vi "Test_API_InitInvalidInputArraySinks_NoLogger.vi"(8 "error in (no error)":errorcluster, 11 "TestCase in":refnum<class "TestLocalLogInstance.lvclass">) -> (0 "error out":errorcluster, 3 "TestCase out":refnum<class "TestLocalLogInstance.lvclass">)   [LabVIEW 2017, in "TestLocalLogInstance.lvclass"]
uses:
  TestLocalLogInstance.lvclass
  Source/Composed Log/Log Sink/Log Sink.lvclass
  Source/Composed Log/LoggerReference/LoggerReference.lvclass/LoggerReference.ctl
  9a0b009a-159a-478b-8bd0-efcaa49947a6.vi
  Source/Composed Log/LoggerReference/Return Aggregate Queues.vi
  Source/Composed Log/LoggerReference/Add Aggregate Log.vi
  9a0b009a-159a-478b-8bd0-efcaa49947a6.vi/8a2c22db-00e5-40c9-a6c7-b08857810732.vi
  Source/Composed Log/LoggerReference/Log.vi
  Source/Composed Log/LoggerReference/Send Add Sink.vi
  Source/Composed Log/LoggerReference/Remove Stale Logs.vi
  Source/Composed Log/Application Logger/Launch Worker Loop.vi
  Source/Composed Log/LoggerReference/Initialize Logger Instance.vi
  Source/Composed Log/LoggerReference/LoggerReference.lvclass
  Source/Composed Log/IErrorFormat/IErrorFormat.lvclass
  <vilib>/addons/_JKI Toolkits/VI Tester/TestCase.llb/TestCase.lvclass
  C:/Program Files (x86)/National Instruments/LabVIEW 2017/vi.lib/addons/_JKI Toolkits/VI Tester/TestCase.llb/TestCase.lvclass
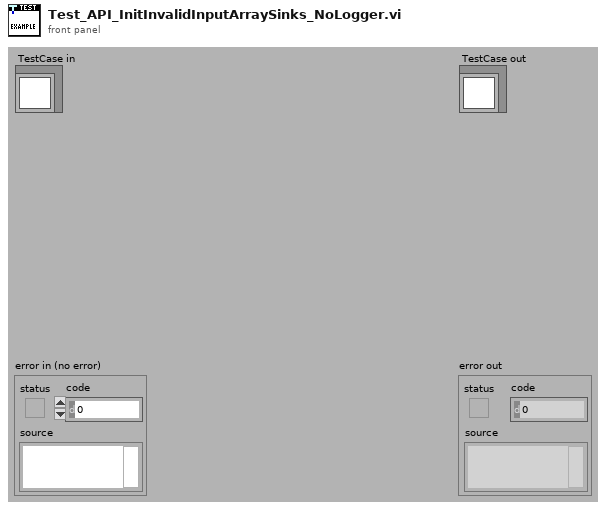
[diagram p1: front panel]
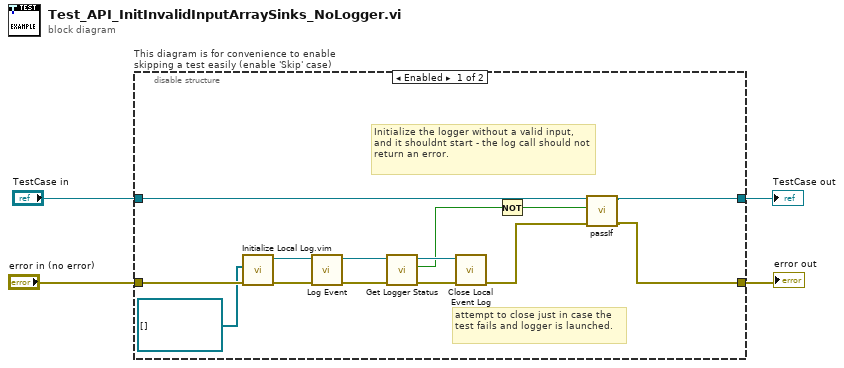
[diagram p0: block diagram]
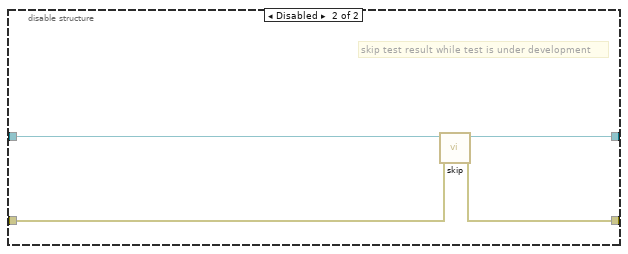
[diagram p2: hidden frame]
diagram:
  n1 = disable-structure "This diagram is for convenience to enable skipping a test easily (enable 'Skip' case)" shown="Enabled" {
    disable-tunnel: "TestCase in" -> [w12 w22]
    disable-tunnel: [w11 w20] -> w1
    disable-tunnel: [w14 w21] -> w3
    disable-tunnel: "error in (no error)" -> [w18 w19]
    frame Enabled {
      # "attempt to close just in case the test fails and logger is launched."
      # "Initialize the logger without a valid input, and it shouldnt start - the log call should not return an error."
      n2 = call "Initialize Local Log.vim"("error in (no error)"=w18, "Startup Sink(s)"=refnum<class "Log Sink.lvclass">[] [] ("Log Sink")) -> ("error out"=w17:errorcluster, "Log Instance Reference"=w16:refnum<class "LoggerReference.lvclass">)  [unwired: 7 in, 1 out]
      n3 = call "Log Event.vi"("error in (no error)"=w17, "Log Instance"=w16) -> ("error out"=w9:errorcluster, "Log Instance Out"=w10:refnum<class "LoggerReference.lvclass">)  [unwired: 8 in]
      n4 = call "Get Logger Status.vi"("error in (no error)"=w9, "LoggerReference in"=w10) -> ("error out"=w7:errorcluster, "Logger Instantiated?"=w6:bool, "LoggerReference out"=w8:refnum<class "LoggerReference.lvclass">)  [unwired: 6 in, 1 out]
      n5 = call "Close Local Event Log.vi"("error in (no error)"=w7, "Log Instance"=w8) -> ("error out"=w13:errorcluster)  [unwired: 9 in]
      n6 = Not(x=w6) -> (.not. x?=w5:bool)
      n7 = call-dynamic "passIf.vi"("error in (no error)"=w13, "pass"=w5, "TestCase in"=w12) -> ("error out"=w14:errorcluster, "TestCase out"=w11:refnum<class "TestLocalLogInstance.lvclass">)  [unwired: 7 in]
    }
    frame Disabled {
      # "skip test result while test is under development"
      n8 = call <vilib>:"skip.vi"("error in (no error)"=w19, "TestCase in"=w22) -> ("error out"=w21:errorcluster, "TestCase out"=w20:refnum<class "TestLocalLogInstance.lvclass">)  [unwired: 8 in]
    }
  }
  "error out" <- w3
  "TestCase out" <- w1
